vi "front panel state ajg.vi"(8 "error in (no error)":errorcluster, 9 "show front panel":bool, 11 "VI in":refnum<vi>) -> (0 "error out":errorcluster)   [LabVIEW 2020]
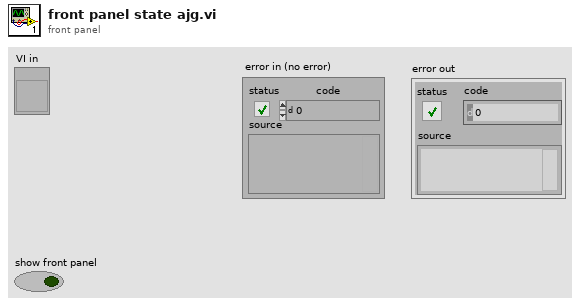
[diagram p1: front panel]
types:
  T1 = enum32{"Invalid", "Standard", "Closed", "Hidden", "Minimized", "Maximized"}
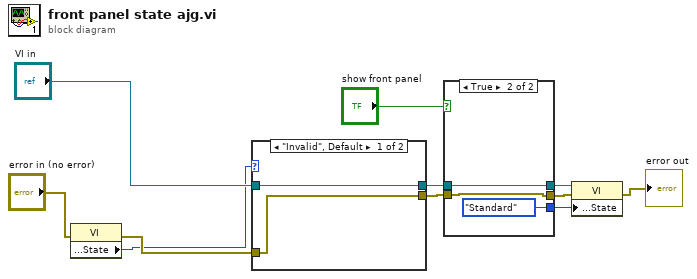
[diagram p0: block diagram]
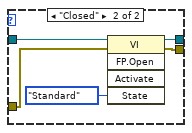
[diagram p2: hidden frame]
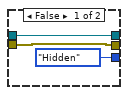
[diagram p3: hidden frame]
diagram:
  n1 = property class="VI"(error in="error in (no error)") -> (error out=w2:errorcluster, "Front Panel Window:State"=w1:T1)  [unwired: 1 in, 1 out]
  n2 = case shown="\"Invalid\", Default" w1 {
    tunnel: "VI in" -> [w13 w18]
    tunnel: [w13 w17] -> w10
    tunnel: w2 -> [w12 w16]
    tunnel: [w12 w15] -> w6
    frame "Invalid", Default {
    }
    frame "Closed" {
      n3 = invoke class="VI" method="FP.Open"(reference=w18, error in=w16, "State"=T1."Standard") -> (reference out=w17:refnum<vi>, error out=w15:errorcluster)  [unwired: 2 in, 3 out]
    }
  }
  n4 = case shown="True" "show front panel" {
    tunnel: w10 -> [w20 w23]
    tunnel: [T1."Hidden" ("State") T1."Standard" ("State")] -> w8
    tunnel: [w20 w23] -> w11
    tunnel: w6 -> [w19 w22]
    tunnel: [w19 w22] -> w5
    frame False {
    }
    frame True {
    }
  }
  n5 = property class="VI"(reference=w11, error in=w5, "Front Panel Window:State"=w8) -> (error out=→"error out":errorcluster)  [unwired: 1 out]
